vi "Set Plot visiblity.vi"(8 "error in (no error)":errorcluster, 10 "Plot visibility":T1[](array[typedef]), 11 "Graph_refs":T2) -> (0 "error out":errorcluster)   [LabVIEW 2018]
uses:
  Scope/controls/Graph_references.ctl
  Scope/controls/graph_controls.ctl
  Scope/controls/Plot visibility.ctl
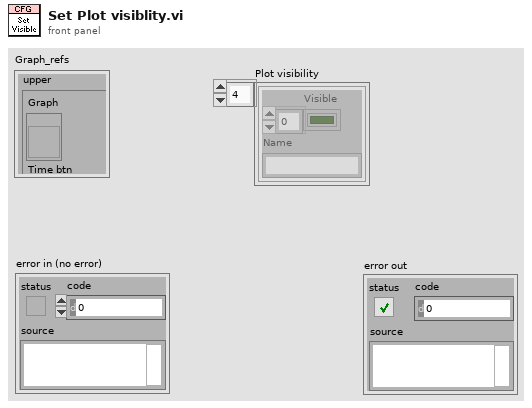
[diagram p1: front panel]
types:
  T1 = typedef "Plot visibility.ctl" = cluster{"Visible":bool[], "Name":string}
  T2 = typedef "Graph_references.ctl" = cluster{"upper":T3, "lower":T3, "Freq graph":refnum<vi>, "Adaptive FF graph":refnum<vi>}
  T3 = typedef "graph_controls.ctl" = cluster{"Graph":refnum<vi>, "Time btn":refnum<vi>, "Amplitude btn":refnum<vi>, "Chart":refnum<vi>}
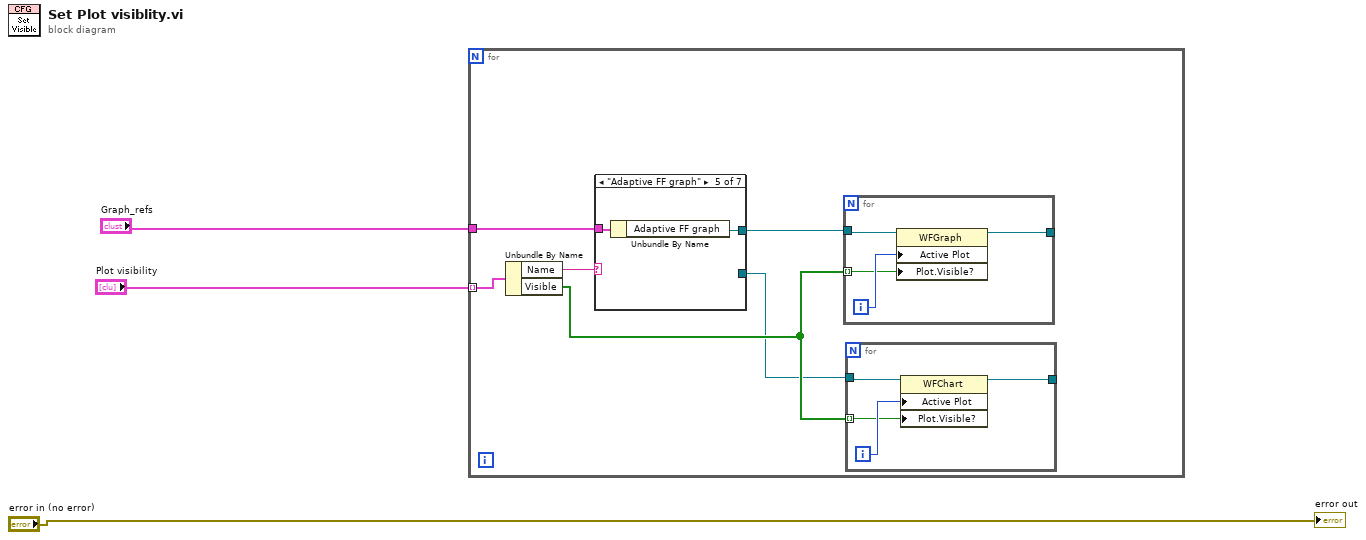
[diagram p0: block diagram]
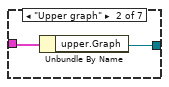
[diagram p3: hidden frame]
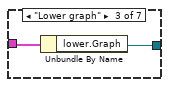
[diagram p4: hidden frame]
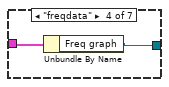
[diagram p5: hidden frame]
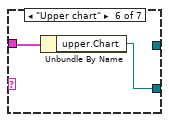
[diagram p6: hidden frame]
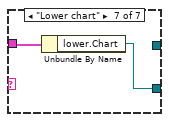
[diagram p7: hidden frame]
diagram:
  n1 = for {
    tunnel: "Plot visibility" -> [w9] mode=indexing
    tunnel: "Graph_refs" -> [w7]
    n2 = Unbundle By Name(w9) -> ("Name"=w8:string, "Visible"=w5:bool[])
    n3 = case shown="\"Adaptive FF graph\"" w8 {
      tunnel: w7 -> [_ w19 w21 w23 w25 w27 w29]
      tunnel: [_ w18 w20 w22 w24 _ _] -> w6
      tunnel: [_ _ _ _ _ w26 w28] -> w4
      frame Default {
      }
      frame "Upper graph" {
        n4 = Unbundle By Name(w19) -> ("upper.Graph"=w18:refnum<vi>)
      }
      frame "Lower graph" {
        n5 = Unbundle By Name(w21) -> ("lower.Graph"=w20:refnum<vi>)
      }
      frame "freqdata" {
        n6 = Unbundle By Name(w23) -> ("Freq graph"=w22:refnum<vi>)
      }
      frame "Adaptive FF graph" {
        n7 = Unbundle By Name(w25) -> ("Adaptive FF graph"=w24:refnum<vi>)
      }
      frame "Upper chart" {
        n8 = Unbundle By Name(w27) -> ("upper.Chart"=w26:refnum<vi>)
      }
      frame "Lower chart" {
        n9 = Unbundle By Name(w29) -> ("lower.Chart"=w28:refnum<vi>)
      }
    }
    n10 = for {
      tunnel: w6 -> [w17]
      tunnel: [w15] -> _
      tunnel: w5 -> [w14] mode=indexing
      i -> [w16]
      n11 = property on="Property Node" class="WFGraph"(reference=w17, "Active Plot"=w16, "Plot.Visible?"=w14) -> (reference out=w15:refnum<vi>)  [unwired: 1 in, 1 out]
    }
    n12 = for {
      tunnel: w4 -> [w10]
      tunnel: [w12] -> _
      tunnel: w5 -> [w11] mode=indexing
      i -> [w13]
      n13 = property on="Property Node" class="WFChart"(reference=w10, "Active Plot"=w13, "Plot.Visible?"=w11) -> (reference out=w12:refnum<vi>)  [unwired: 1 in, 1 out]
    }
  }
  "error out" <- "error in (no error)"
